vi "Random Number Generator.vi"() -> ()   [LabVIEW 2014]
doc: "This Vi generates a random number from a geiger counter output. You tell the VI what bit number you want and it outputs this number in decimal form."
uses:
  <vilib>/imath/engines/lvmath/Plug In/_Char/NIMS_CH_character datatype.ctl
  <vilib>/imath/engines/lvmath2/RunTimeEngine/Managers/WorkSpace/UID Generator.vi
  <vilib>/imath/engines/lvmath2/RunTimeEngine/RunTimeType/NIMS_RunTimeType_From StrictType (excl LVString).vi
  <instcachedir>/0/NIMS_RunTimeType_From StrictType (excl LVString)_15A5391EEA9C4AACB9955AC755B83D29.lvgen/NIMS_RunTimeType_From StrictType (excl LVString)_15A5391EEA9C4AACB9955AC755B83D29_000.vi
  <vilib>/imath/engines/lvmath2/RunTimeEngine/LocalVariableDefStatement/MC_LocalVariableDefStatement_Display.vi
  <vilib>/imath/engines/lvmath2/RunTimeEngine/Managers/SymbolTable/Clear UID.vi
  <vilib>/imath/engines/lvmath2/RunTimeEngine/NodeEndStatement/NIMS_NodeEndStatement_Output.vi
  <instcachedir>/0/NIMS_NodeEndStatement_Output_53EC0D466D134D7ABD903AC30B43404B.lvgen/NIMS_NodeEndStatement_Output_53EC0D466D134D7ABD903AC30B43404B_012.vi
  <vilib>/imath/engines/lvmath2/RunTimeEngine/ErrorHandling/NIMS_Finalize Error.vi
  <vilib>/imath/engines/lvmath2/RunTimeEngine/VariableToken/Support/NIMS_Vector Boolean Index to I32 Index.vi
  <vilib>/imath/engines/lvmath2/RunTimeEngine/IndexRead/NIMS V(V).vi
  <instcachedir>/0/NIMS V(V)_298D9CB7BFEB42B8BC8D9C3C28AE8C70.lvgen/NIMS V(V)_298D9CB7BFEB42B8BC8D9C3C28AE8C70_000.vi
  <vilib>/imathl/engines/lvmath/Functions/Error Handling/Create Error.vi
  <vilib>/imath/engines/lvmath2/RunTimeEngine/BuiltInFunctions/num_to_str/NIMS_num_to_str(GRowV,I32).vi
  <instcachedir>/0/NIMS_num_to_str(GRowV,I32)_6C1A87207DE5453397F3BF129F24C119.lvgen/NIMS_num_to_str(GRowV,I32)_6C1A87207DE5453397F3BF129F24C119_000.vi
  <vilib>/imath/engines/lvmath/Plug In/_Char/NIMS_CH_String to Character Array.vi
  <instcachedir>/0/NIMS_RunTimeType_From StrictType (excl LVString)_15A5391EEA9C4AACB9955AC755B83D29.lvgen/NIMS_RunTimeType_From StrictType (excl LVString)_15A5391EEA9C4AACB9955AC755B83D29_001.vi
  <vilib>/imath/engines/lvmath2/RunTimeEngine/ErrorHandling/NIMS_Error From Error Code.vi
  <vilib>/imath/engines/lvmath2/RunTimeEngine/BuiltInFunctions/is_space/NIMS_is_space(string).vi
  <vilib>/imath/engines/lvmath2/RunTimeEngine/IndexReplace/NIMS V(V)=V.vi
  <instcachedir>/0/NIMS V(V)=V_1E3A7F7F615C46EF9FDD71F29C66FCF8.lvgen/NIMS V(V)=V_1E3A7F7F615C46EF9FDD71F29C66FCF8_000.vi
  <vilib>/imath/engines/lvmath/Plug In/_Char/NIMS_CH_Character 2D to String 1D.vi
  <vilib>/imath/engines/lvmath2/RunTimeEngine/BuiltInFunctions/bin_to_dec/NIMS_bin_to_dec.vi
  <instcachedir>/0/NIMS_NodeEndStatement_Output_53EC0D466D134D7ABD903AC30B43404B.lvgen/NIMS_NodeEndStatement_Output_53EC0D466D134D7ABD903AC30B43404B_005.vi
  <vilib>/imath/engines/lvmath2/RunTimeEngine/Managers/SymbolTable/NIMS_WorkSpace.lvlib
panel:
  out "Gauge":dbl(knob) scale=0.0..100.0
  out "Random Number":cluster{"Random Number":dbl[]}
  in  "Binary Digits":cluster{"Num Digits":dbl}
  out "Array":i32[](array[numeric])
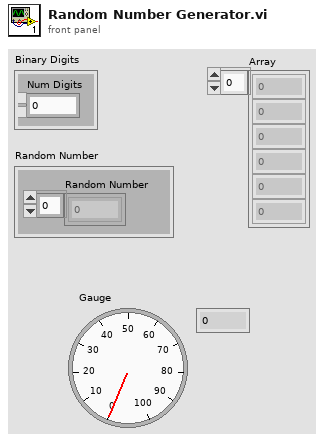
[diagram p1: front panel]
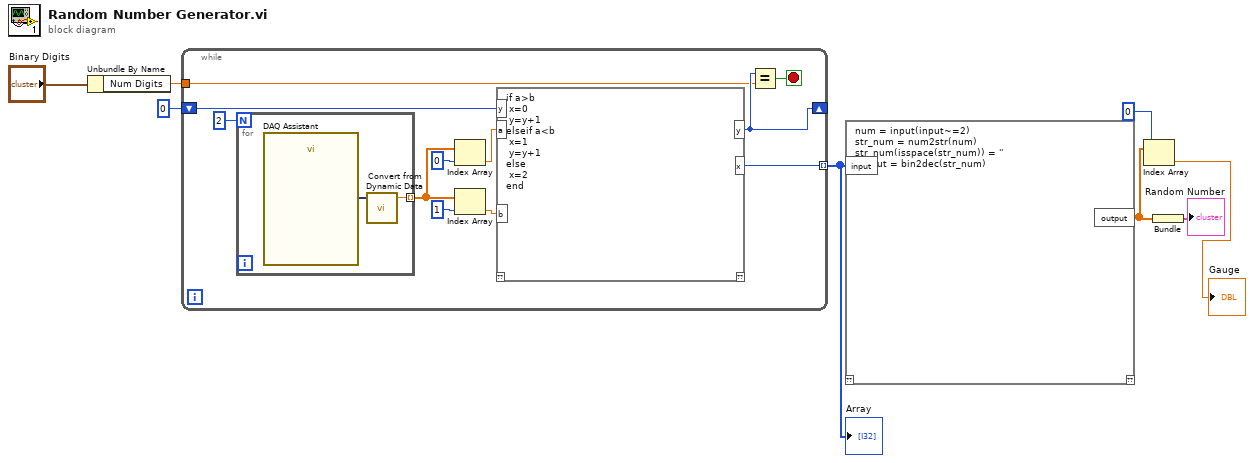
[diagram p0: block diagram]
diagram:
  n1 = Unbundle By Name("Binary Digits") -> ("Num Digits"=w5:dbl)
  n2 = while {
    shift-right: [w12] -> _
    shift-left: 0 -> [w13]
    tunnel: w5 -> [w11]
    tunnel: [w9] -> w7 mode=indexing
    stop <- w10 stop-if-true
    n3 = for {
      N: 2 -> [_]
      tunnel: [w150] -> w18 mode=indexing
      n4 = call "DAQ Assistant"() -> ("data"=w151:dynamicdata)  [unwired: 17 in, 2 out]
      n5 = call "Convert from Dynamic Data"("Dynamic Data Type"=w151) -> ("Scalar"=w150:dbl)  [unwired: 3 in]
    }
    n6 = Index Array(array=w18, index=0) -> (element=w15:dbl)
    n7 = Index Array(array=w18, index=1) -> (element=w14:dbl)
    n8 = mathscript code="if a>b\n x=0\n y=y+1\nelseif a<b\n x=1\n y=y+1\nelse\n x=2\nend"("a"=w15, "b"=w14, "y"=w13) -> ("x"=w9:i32, "y"=w12:i32)  [unwired: 1 in, 1 out]
    n9 = Equal?(x=w12, y=w11) -> (x = y?=w10:bool)
  }
  "Array" <- w7
  n10 = mathscript code="num = input(input~=2)\nstr_num = num2str(num)\nstr_num(isspace(str_num)) = ''\noutput = bin2dec(str_num)"("input"=w7) -> ("output"=w3:dbl[])  [unwired: 1 in, 1 out]
  n11 = Index Array(array=w3, index=0) -> (element=→"Gauge":dbl)
  n12 = Bundle("output"=w3) -> (→"Random Number":cluster{"output":dbl[]})  [unwired: 1 in]
